vi "数据表比对1表格对比.vi"(8 "error in (no error)":errorcluster, 9 "table输入 2":string(combo), 11 "table输入":string(combo)) -> (0 "error out":errorcluster, 2 "待发送第一条数据":string[](array[string]), 3 "待发送数据":string[][](table), 4 "获取有效数据":string[][](array[string]))   [LabVIEW 2016]
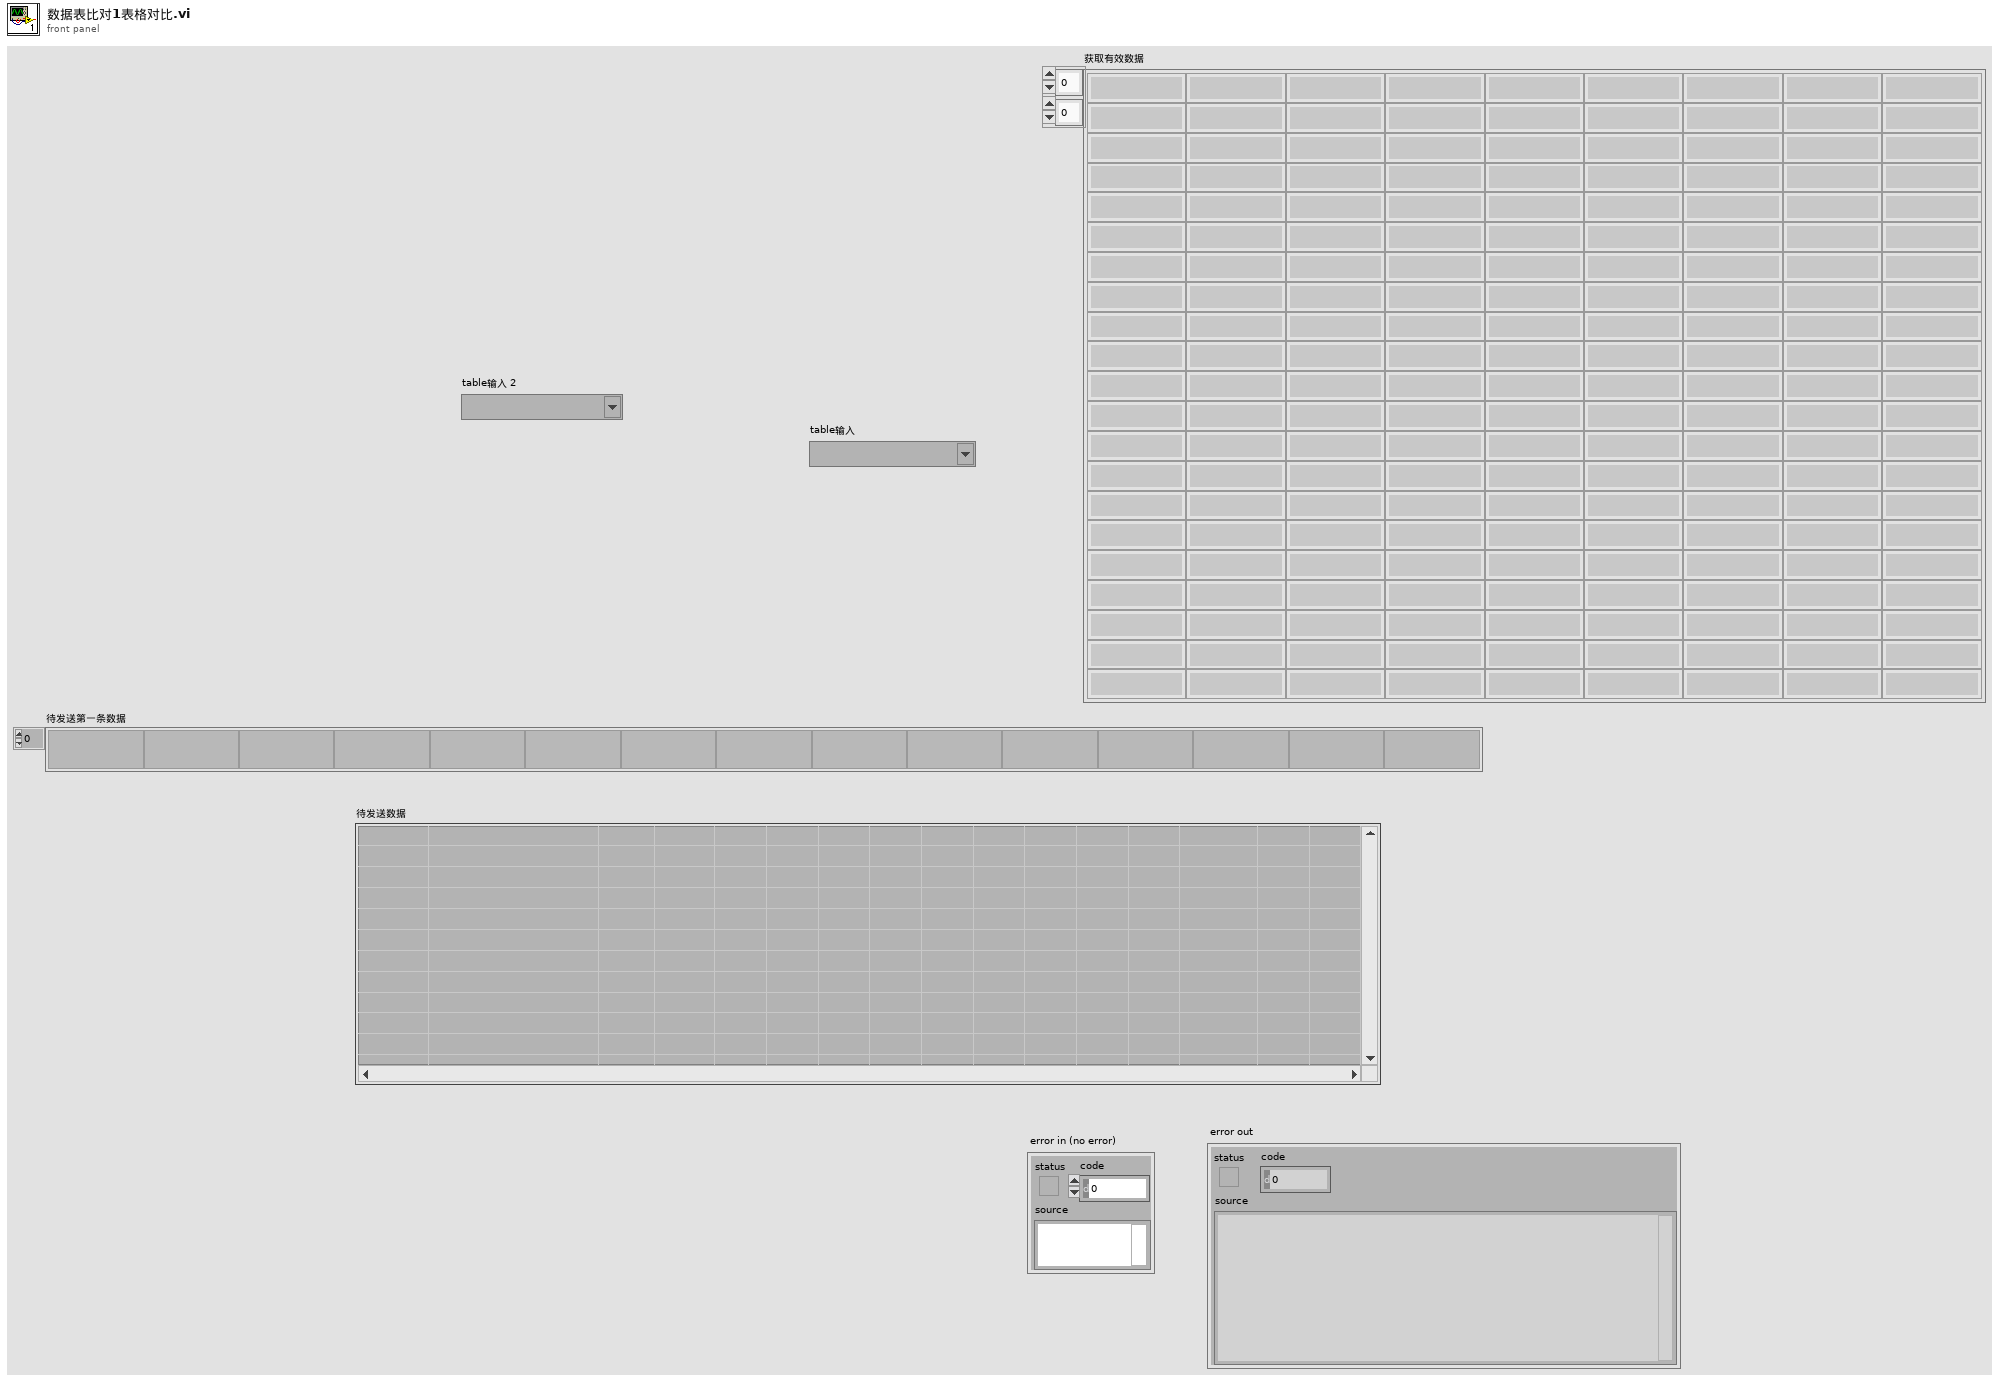
[diagram p1: front panel]
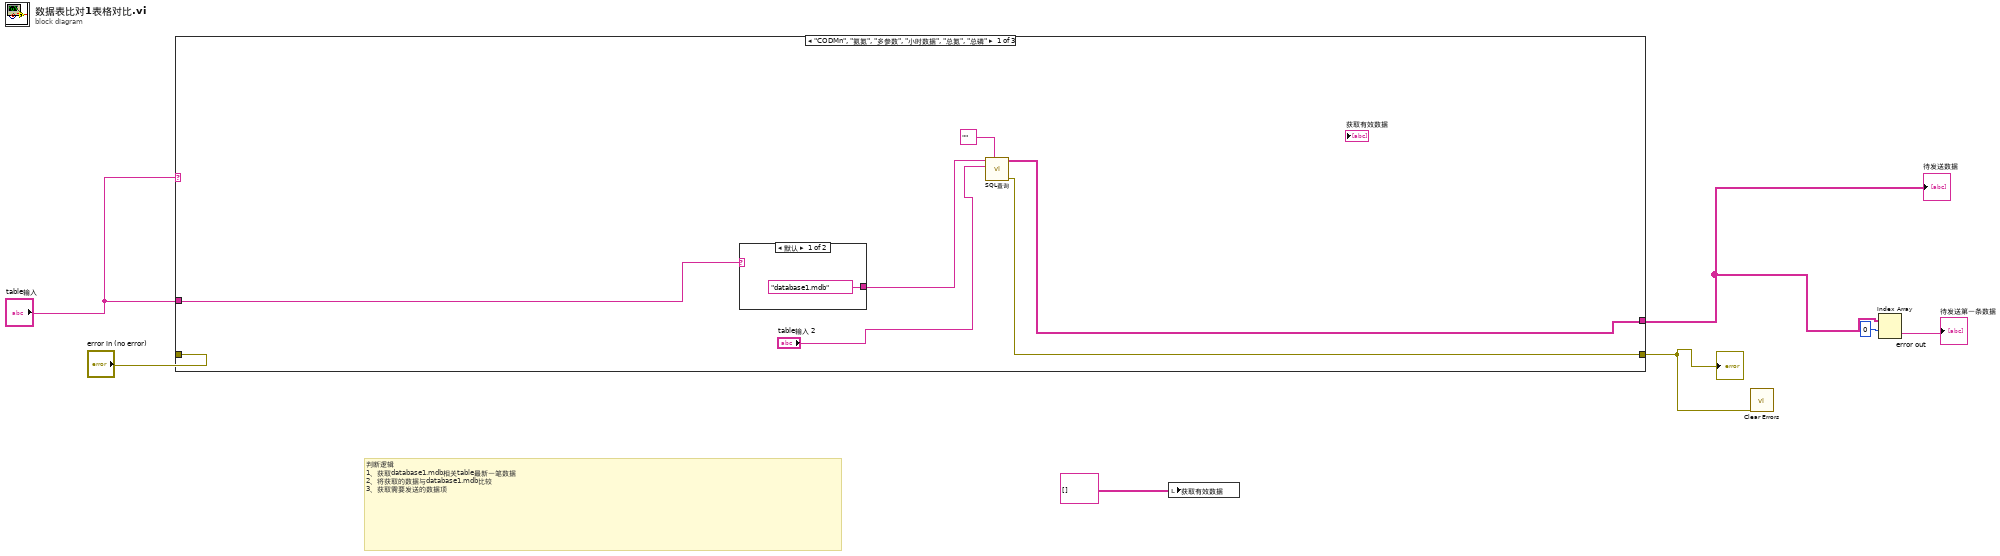
[diagram p0: block diagram]
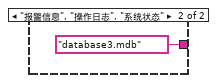
[diagram p2: hidden frame]
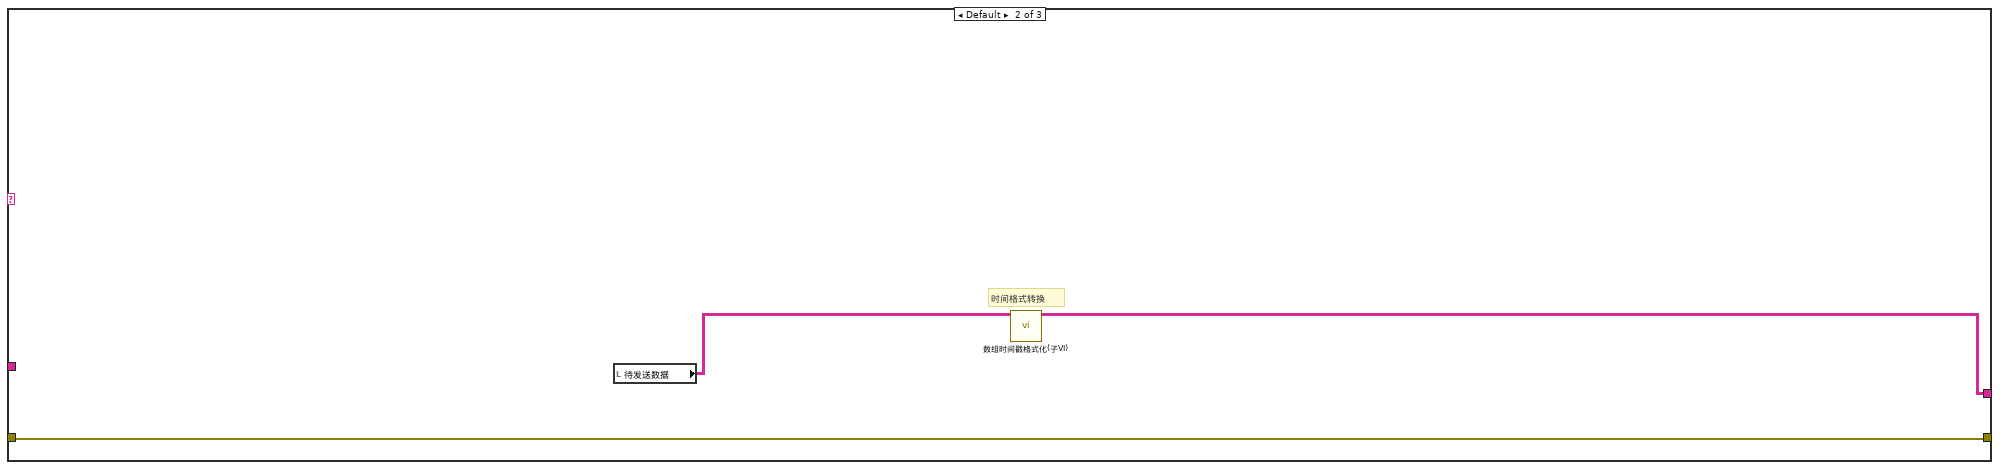
[diagram p3: hidden frame]
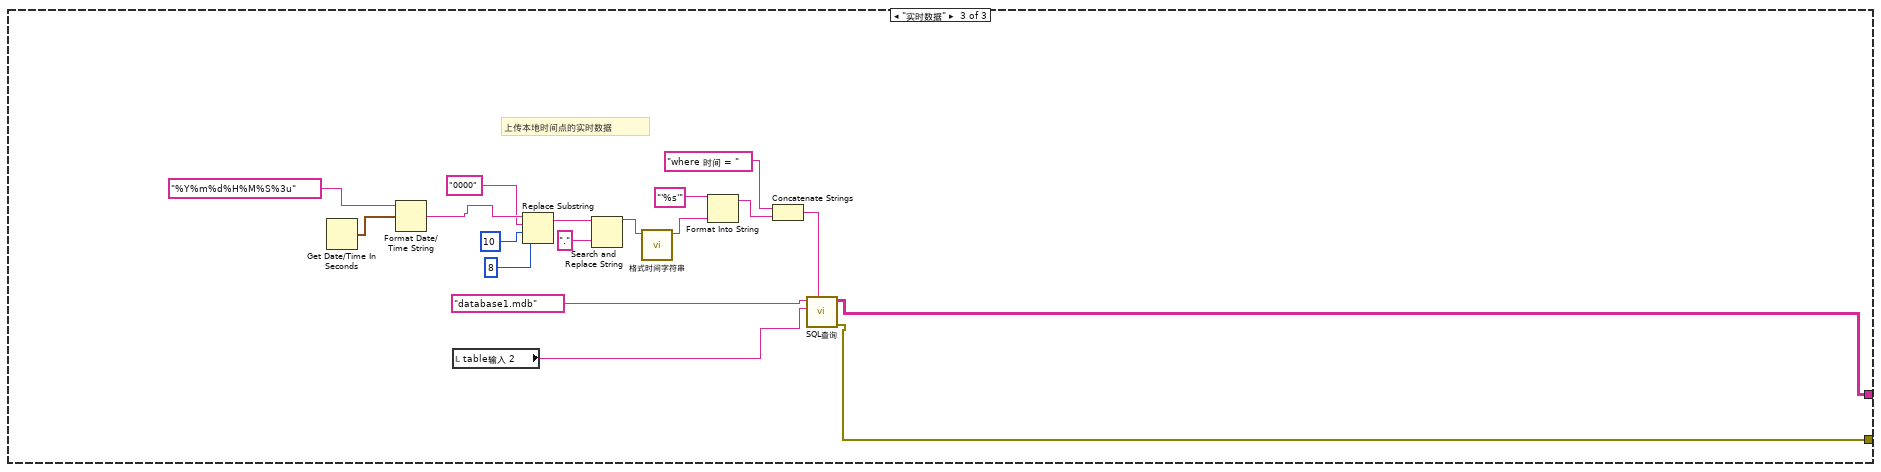
[diagram p4: hidden frame]
diagram:
  # "判断逻辑\n1、获取database1.mdb相关table最新一笔数据\n2、将获取的数据与database1.mdb比较\n3、获取需要发送的数据项"
  n1 = case shown="\"CODMn\", \"氨氮\", \"多参数\", \"小时数据\", \"总氮\", \"总磷\"" "table输入" {
    tunnel: "error in (no error)" -> [_ w18 _]
    tunnel: [w10 w18 w26] -> w5
    tunnel: [w9 w16 w27] -> w1
    tunnel: "table输入" -> [w13 _ _]
    frame "CODMn", "氨氮", "多参数", "小时数据", "总氮", "总磷" {
      n2 = case shown="默认" w13 {
        tunnel: ["database1.mdb" ("database") "database3.mdb" ("database")] -> w12
        frame Default {
        }
        frame "报警信息", "操作日志", "系统状态" {
        }
      }
      n3 = call "SQL查询.vi"("condition"="", "table输入"="table输入 2", "database"=w12) -> ("error out"=w10:errorcluster, "data"=w9:string[][])  [unwired: 7 in]
    }
    frame Default {
      # "时间格式转换"
      n4 = local read "待发送数据"() -> (w17:string[][])
      n5 = call "数组时间戳格式化(子VI).vi"("待发送数据输入"=w17) -> ("待发送数据输出"=w16:string[][])  [unwired: 10 in]
    }
    frame "实时数据" {
      # "上传本地时间点的实时数据"
      n6 = Get Date/Time In Seconds() -> (seconds since 1Jan1904=w32:timestamp)
      n7 = Format Date/Time String(time format string (%c)="%Y%m%d%H%M%S%3u" ("时间格式字符串(%c)"), seconds (now)=w32) -> (date/time string=w25:string)  [unwired: 1 in]
      n8 = local read "table输入 2"() -> (w28:string)
      n9 = Replace Substring(2:8 ("长度（子字符串长度）"), 3:10 ("偏移量(0)"), 4:"0000" ("子字符串(\"\")"), 5:w25) -> (1:w24:string)  [unwired: 1 out]
      n10 = Search and Replace String(input string=w24, search string="." ("搜索字符串")) -> (result string=w20:string)  [unwired: 6 in, 3 out]
      n11 = call "格式时间字符串.vi"("字符串"=w20) -> ("连接的字符串"=w19:string)  [unwired: 10 in]
      n12 = Format Into String(format string="'%s'" ("初始字符串"), w19) -> (resulting string=w35:string)  [unwired: 2 in, 1 out]
      n13 = Concatenate Strings("where 时间 = " ("condition"), w35) -> (w30:string)
      n14 = call "SQL查询.vi"("condition"=w30, "table输入"=w28, "database"="database1.mdb") -> ("error out"=w26:errorcluster, "data"=w27:string[][])  [unwired: 7 in]
    }
  }
  "待发送数据" <- w1
  "error out" <- w5
  n15 = local write "获取有效数据"(string[][] []) -> ()
  n16 = call <vilib>:"Clear Errors.vi"("error in (no error)"=w5) -> ()  [unwired: 5 in, 2 out]
  n17 = Index Array(array=w1, index (row)=0 ("索引 (行)")) -> (element=→"待发送第一条数据":string[])  [unwired: 1 in]
